vi "ExGetParamInfo .vi"() -> ()   [LabVIEW 2010]
uses:
  Users/Public/Documents/SItoolkit/LabVIEW/Examples2010_5_0_0_0/Fast Examples/Open-Close Hardware/CamHandle.vi
panel:
  out "default value":dbl
  out "current value":dbl
  out "num of elements":dbl
  in  "parameter ID":u32
  out "error out":errorcluster
  in  "error in (no error)":errorcluster
  # "121 - vertical speed\n45 - adc speed"
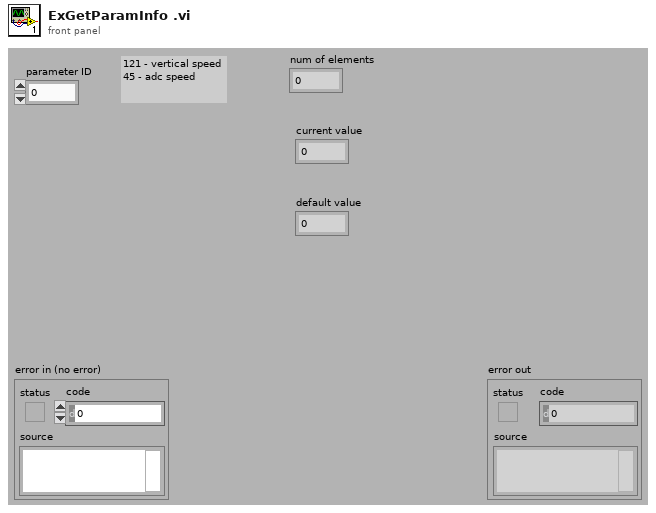
[diagram p1: front panel]
types:
  T1 = cluster{"Param ID":u32, "Avail Flag":u8, "Current Value":dbl, "Default Value":dbl, "Min Value":dbl, "Max Value":dbl, "Increment":dbl, "Data Type":u32, "Access Type":u32, "Bit Used Flag":u32, "Number of Enums":u32, "Description":string}
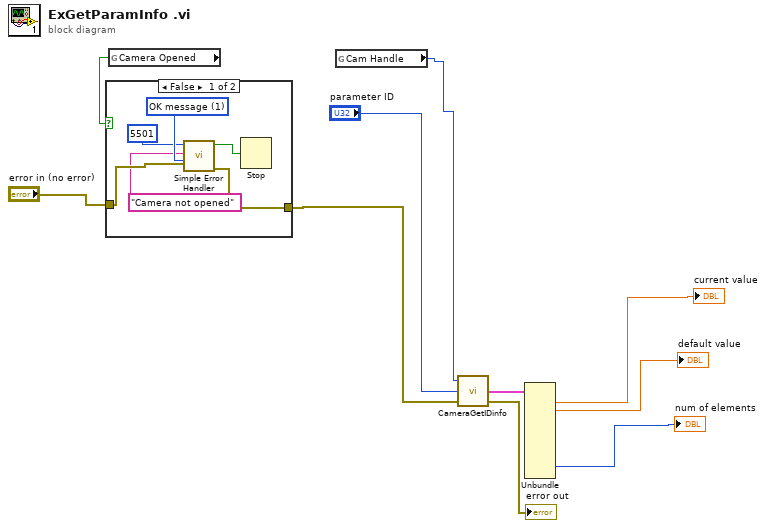
[diagram p0: block diagram]
diagram:
  n1 = global read "CamHandle.vi" "Camera Opened"() -> (w10:bool)
  n2 = case shown="False" w10 {
    tunnel: "error in (no error)" -> [w15 w17]
    tunnel: [w14 w17] -> w7
    frame False {
      w16 = u16 1 items=["no dialog", "OK message", "continue or stop message"] ("type of dialog (OK msg:1)")
      n3 = call <vilib>:"Simple Error Handler.vi"("error code (no error:0)"=5501, "error source (\" \")"="Camera not opened", "type of dialog (OK msg:1)"=w16, "error in (no error)"=w15) -> ("error?"=w12:bool, "error out"=w14:errorcluster)  [unwired: 1 in, 3 out]
      n4 = Stop(stop? (T)=w12) -> ()
    }
    frame True {
    }
  }
  n5 = global read "CamHandle.vi" "Cam Handle"() -> (w5:u32)
  n6 = call <userlib>:"CameraGetIDinfo.vi"("error in"=w7, "Param ID"="parameter ID", "Camera handle"=w5) -> ("error out"=→"error out":errorcluster, "Param ID Information"=w8:T1)  [unwired: 1 out]
  n7 = Unbundle(w8) -> ("Current Value"=→"current value":dbl, "Default Value"=→"default value":dbl, "Number of Enums"=→"num of elements":u32)  [unwired: 9 out]
